vi "Command Create (2 parameters).vi"(5 "Parameter 2":i64, 7 "Parameter 1":i64, 9 "Command Mode":enum16{"Write", "Read"}(ring), 10 "Command Type":T1(ring), 11 "Command Name":string) -> (2 "Command":string)   [LabVIEW 2017, in "Roboteq Controller KBL1xxx.lvlib"]
uses:
  <instrlib>/Roboteq Controller KBL1xxx/Roboteq Controller KBL1xxx.lvlib
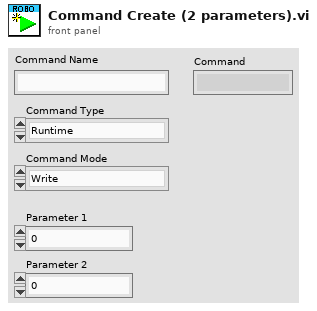
[diagram p1: front panel]
types:
  T1 = enum16{"Runtime", "Configuration", "Maintenance"}
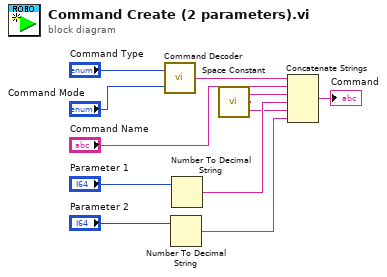
[diagram p0: block diagram]
diagram:
  n1 = call <instrlib>:"Command Decoder.vi"("Command Mode"="Command Mode", "Command Type"="Command Type") -> ("Start symbol"=w8:string)
  n2 = Number To Decimal String(number="Parameter 2") -> (decimal integer string=w2:string)  [unwired: 1 in]
  n3 = Number To Decimal String(number="Parameter 1") -> (decimal integer string=w4:string)  [unwired: 1 in]
  n4 = call <vilib>:"Space Constant.vi"() -> ("String"=w3:string)
  n5 = Concatenate Strings(w8, "Command Name", w3, w4, w3, w2) -> (→"Command":string)
